vi "Get Module Model.vi"(8 "error in (no error)":errorcluster, 11 "Item Ref in":T1 format="%.0x") -> (0 "error out":errorcluster, 2 "Module":T2, 3 "Item Ref out":T3 format="%.0x")   [LabVIEW 2019, in "Scan Engine Custom Device.lvlib"]
uses:
  Scan Engine Custom Device.lvlib
  <vilib>/NI VeriStand/Custom Device API/Custom Device Item Ref.ctl
  Modules.lvlibp/RSI Module/Module Models.ctl
  Modules.lvlibp/1abvi3w/vi.lib/NI VeriStand/Custom Device API/Custom Device Item Ref.ctl
  <vilib>/regexp/Match Regular Expression.xnode
  <vilib>/NI VeriStand/Custom Device API/Custom Device API.lvlib
  Modules.lvlibp/RSI Module/RSI Module.lvclass
  Modules.lvlibp/1abvi3w/vi.lib/NI VeriStand/Custom Device API/Custom Device API.lvlib
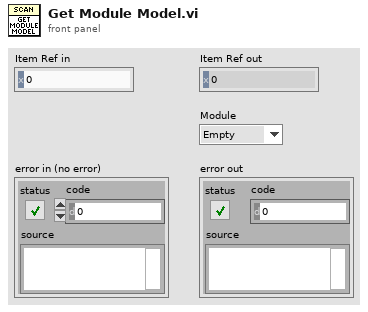
[diagram p1: front panel]
types:
  T1 = typedef "Modules.lvlibp/Custom Device API.lvlib/Custom Device Item Ref.ctl" = u64
  T2 = typedef "Modules.lvlibp/RSI Module.lvclass/Module Models.ctl" = enum16{"Empty", "NI 9201", "NI 9203", "NI 9205", "NI 9206", "NI 9207", "NI 9208", "NI 9209", "NI 9210", "NI 9211", "NI 9212", "NI 9213", "NI 9214", "NI 9215", "NI 9216", "NI 9217", "NI 9219", "NI 9220", "NI 9221", "NI 9222", "NI 9223", "NI 9224", "NI 9225", "NI 9226", "NI 9227", "NI 9228", "NI 9229", "NI 9233", "NI 9234", "NI 9235", "NI 9236", "NI 9237", "NI 9239", "NI 9242", "NI 9244", "NI 9253", "NI 9263", "NI 9264", "NI 9265", "NI 9266", "NI 9269", "NI 9344", "NI 9350", "NI 9375", "NI 9401", "NI 9402", "NI 9403", "NI 9411", "NI 9421", "NI 9422", "NI 9423", "NI 9425", "NI 9426", "NI 9435", "NI 9436", "NI 9437", "NI 9472", "NI 9474", "NI 9475", "NI 9476", "NI 9477", "NI 9478", "NI 9481", "NI 9482", "NI 9485"}
  T3 = typedef "Custom Device API.lvlib/Custom Device Item Ref.ctl" = u64
  T4 = typedef "Custom Device API.lvlib/Custom Device Item Info.ctl" = cluster{"Name":string, "Is Channel":bool, "GUID":string, "Is Waveform":bool}
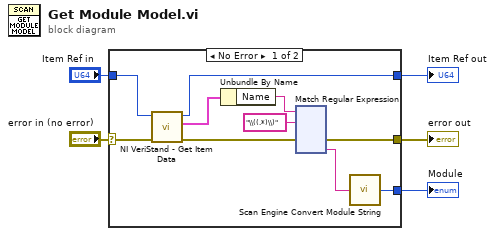
[diagram p0: block diagram]
diagram:
  n1 = case shown="No Error" "error in (no error)" {
    selector: "error in (no error)" -> [w6 w130]
    tunnel: [w15 w129] -> w5
    tunnel: [w14 _] -> w4
    tunnel: [w12 w130] -> w3
    tunnel: "Item Ref in" -> [w11 w129]
    frame No Error {
      n2 = call <vilib>:"NI VeriStand - Get Item Data.vi"("error in (no error)"=w6, "Item Ref in"=w11) -> ("error out"=w8:errorcluster, "Item Info"=w7:T4, "Item Ref out"=w15:T3)  [unwired: 6 in, 1 out]
      n3 = Unbundle By Name(w7) -> ("Name"=w9:string)
      n4 = xnode "Match Regular Expression"("input string"=w9, "regular expression"="\\((.*)\\)", "error in"=w8) -> ("error out"=w12:errorcluster, "submatch 1"=w13:string)  [unwired: 3 in, 4 out]
      n5 = call "Scan Engine Convert Module String.vi"("Module Name"=w13) -> ("Module"=w14:T2)
    }
    frame Error {
    }
  }
  "Item Ref out" <- w5
  "Module" <- w4
  "error out" <- w3
